vi "OneHotEncoder.vi"(8 "error in (no error)":errorcluster caption="entrée d'erreur (pas d'erreur)", 11 "OneHotEncoder":T1={"drop"="None", "sparse"=TRUE, "dtype"="float", "handle_unknown"="error"}) -> (0 "error out":errorcluster, 3 "OneHotEncoder.lvclass":refnum<class "OneHotEncoder.lvclass">)   [LabVIEW 2020]
doc: "Encode categorical features as a one-hot numeric array.\n\nThe input to this transformer should be an array-like of integers or strings, denoting the values taken on by categorical (discrete) features. The features are encoded using a one-hot (aka ‘one-of-K’ or ‘dummy’) encoding scheme. This creates a binary column for each category and returns a sparse matrix or dense array (depending on the sparse parameter)\n\nBy default, the encoder derives the categories based on the unique values in each feature. Alternatively, you can also specify the categories manually.\n\nThis encoding is needed for feeding categorical data to many scikit-learn estimators, notably linear models and SVMs with the standard kernels.\n\nNote: a one-hot encoding of y labels should use a LabelBinarizer instead.\n\n\nParameters\n\n- drop : {‘first’, ‘if_binary’} or a array-like of shape (n_features,), default=None\nSpecifies a methodology to use to drop one of the categories per feature. This is useful in situations where perfectly collinear features cause problems, such as when feeding the resulting data into a neural network or an unregularized regression.\n\nHowever, dropping one category breaks the symmetry of the original representation and can therefore induce a bias in downstream models, for instance for penalized linear classification or regression models.\n\nNone : retain all features (the default).\n\n‘first’ : drop the first category in each feature. If only one category is present, the feature will be dropped entirely.\n\n‘if_binary’ : drop the first category in each feature with two categories. Features with 1 or more than 2 categories are left intact.\n\narray : drop[i] is the category in feature X[:, i] that should be dropped.\n\n- sparse : bool, default=True\nWill return sparse matrix if set True else will return an array.\n\n- dtype : number type, default=np.float\nDesired dtype of output.\n\n- handle_unknown : {‘error’, ‘ignore’}, default=’error’\nWhether to raise an error or ignore if an unknown categorical feature is present during transform (default is to raise). When this parameter is set to ‘ignore’ and an unknown category is encountered during transform, the resulting one-hot encoded columns for this feature will be all zeros. In the inverse transform, an unknown\n\n\nMethods : \n\n\n- Fit : Fit OneHotEncoder to X.\n\nParameters : X : array-like, shape [n_samples, n_features]\n The data to determine the categories of each feature.\n y : None\n Ignored. \n\n\n- Fit Transform : Fit OneHotEncoder to X, then transform X. Equivalent to fit(X).transform(X) but more convenient.\n\nParameters : X : array-like, shape [n_samples, n_features]\n The data to encode.\n y : None\n Ignored. \n\nReturns : X_out : sparse matrix if sparse=True else a 2-d array\n Transformed input.\n\n\n\n- Feature Names : Return feature names for output features.\n\nReturns : output_feature_names : ndarray of shape (n_output_features,)\n Array of feature names.\n\n\n-Transform : Transform X using one-hot encoding.\n\nParameters : X : array-like, shape [n_samples, n_features]\n The data to encode.\n\nReturns : X_out : sparse matrix if sparse=True else a 2-d array\n Transformed input."
uses:
  OneHotEncoder.lvclass
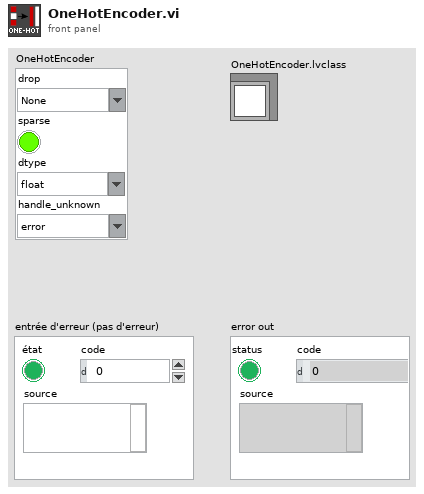
[diagram p1: front panel]
types:
  T1 = cluster{"drop":string, "sparse":bool, "dtype":string, "handle_unknown":string}
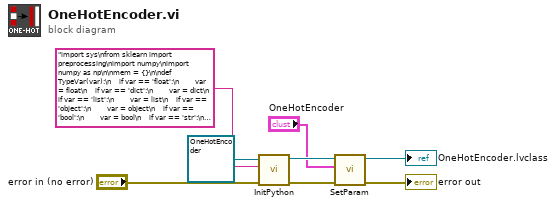
[diagram p0: block diagram]
diagram:
  n1 = call-dynamic "InitPython.vi"("error in (no error)"="error in (no error)", "Python Instruction"="import sys\nfrom sklearn import preprocessing\nimport numpy\nimport numpy as np\n\nmem = {}\n\ndef TypeVar(var):\n    if var == 'float':\n        var = float\n    if var == 'dict':\n        var = dict\n    if var == 'list':\n        var = list\n    if var == 'object':\n        var = object\n    if var == 'bool':\n        var = bool\n    if var == 'str':\n        var = str\n    if var == 'int':\n        var = int\n    return var\n\ndef OneHotEncoder_Fit(categories, drop, sparse, dtype, handle_unknown, X, y):\n    X = eval(X)\n    dtype = TypeVar(dtype)\n    if drop == 'None':\n        drop = None\n    if y == 'None' or y == '':\n        y = None\n    else:\n        y = eval(y)\n    try:\n        OneHotEncoder = preprocessing.OneHotEncoder(categories, drop, sparse, dtype, handle_unknown).fit(X, y)\n        mem['FitOneHotEncoder'] = OneHotEncoder\n        return str('OK')\n    except:\n        erreur = sys.exc_info()\n        typerr = u\"%s\" % (erreur[0])\n        typerr = typerr[typerr.find(\"'\")+1:typerr.rfind(\"'\")]\n        msgerr = u\"%s\" % (erreur[1])\n        message = str('/!\\\\ {0} : {1}'. format(typerr,msgerr))\n        return message \n    \ndef OneHotEncoder_FitTransform(categories, drop, sparse, dtype, handle_unknown, X, y):\n    X = eval(X)\n    dtype = TypeVar(dtype)\n    if drop == 'None':\n        drop = None\n    if y == 'None' or y == '':\n        y = None\n    else:\n        y = eval(y)\n    try:\n        OneHotEncoder = preprocessing.OneHotEncoder(categories, drop, sparse, dtype, handle_unknown).fit_transform(X, y)\n        dtype_func = type(OneHotEncoder)\n        if dtype_func == numpy.ndarray:\n            OneHotEncoder = OneHotEncoder.tolist()\n            return str(OneHotEncoder) \n        else:\n            Mat = OneHotEncoder.tocoo()\n            return str(list(zip(Mat.row, Mat.col, Mat.data)))\n    except:\n        erreur = sys.exc_info()\n        typerr = u\"%s\" % (erreur[0])\n        typerr = typerr[typerr.find(\"'\")+1:typerr.rfind(\"'\")]\n        msgerr = u\"%s\" % (erreur[1])\n        message = str('/!\\\\ {0} : {1}'. format(typerr,msgerr))\n        return message \n\ndef OneHotEncoder_Transform(categories, drop, sparse, dtype, handle_unknown, X, y):\n    X = eval(X)\n    dtype = TypeVar(dtype)\n    if drop == 'None':\n        drop = None\n    if y == 'None' or y == '':\n        y = None\n    else:\n        y = eval(y)\n    try:\n        OneHotEncoder = mem['FitOneHotEncoder'].transform(X)\n        dtype_func = type(OneHotEncoder)\n        if dtype_func == numpy.ndarray:\n            OneHotEncoder = OneHotEncoder.tolist()\n            return str(OneHotEncoder) \n        else:\n            Mat = OneHotEncoder.tocoo()\n            return str(list(zip(Mat.row, Mat.col, Mat.data)))\n    except:\n        erreur = sys.exc_info()\n        typerr = u\"%s\" % (erreur[0])\n        typerr = typerr[typerr.find(\"'\")+1:typerr.rfind(\"'\")]\n        msgerr = u\"%s\" % (erreur[1])\n        message = str('/!\\\\ {0} : {1}'. format(typerr,msgerr))\n        return message\n\ndef OneHotEncoder_Feature_Names(categories, drop, sparse, dtype, handle_unknown, X, y):\n    dtype = eval(dtype)\n    if drop == 'None':\n        drop = None\n    if y == 'None' or y == '':\n        y = None\n    else:\n        y = eval(y)\n    try:\n        OneHotEncoder_feature_names = mem['FitOneHotEncoder'].get_feature_names()\n        return str(OneHotEncoder_feature_names)\n    except:\n        erreur = sys.exc_info()\n        typerr = u\"%s\" % (erreur[0])\n        typerr = typerr[typerr.find(\"'\")+1:typerr.rfind(\"'\")]\n        msgerr = u\"%s\" % (erreur[1])\n        message = str('/!\\\\ {0} : {1}'. format(typerr,msgerr))\n        return message", "Scikit-learn en entrée"=refnum<class "OneHotEncoder.lvclass"> refnum ("OneHotEncoder.lvclass")) -> ("error out"=w5:errorcluster, "Scikit-learn en sortie"=w4:refnum<class "OneHotEncoder.lvclass">)  [unwired: 7 in]
  n2 = call-dynamic "SetParam.vi"("error in (no error)"=w5, "OneHotEncoder"="OneHotEncoder", "OneHotEncoder.lvclass"=w4) -> ("error out"=→"error out":errorcluster, "OneHotEncoder.lvclass"=→"OneHotEncoder.lvclass":refnum<class "OneHotEncoder.lvclass">)  [unwired: 7 in]
